vi "Set Sender.vi"(10 "Sender":string, 11 "Message":refnum<class "Message.lvclass">) -> (3 "Message":refnum<class "Message.lvclass">)   [LabVIEW 2017, in "LapDog.Messaging.v3.lvlib" / "Message.lvclass"]
uses:
  Message.lvclass
  Message.lvclass/Message.ctl
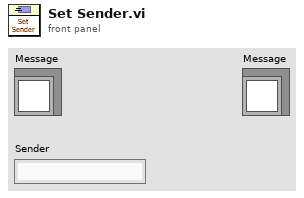
[diagram p1: front panel]
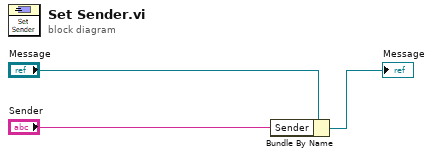
[diagram p0: block diagram]
diagram:
  n1 = Bundle By Name(cluster="Message", "Sender"="Sender") -> (→"Message":refnum<class "Message.lvclass">)
